vi "SCLN_TCPWritewithSize.vi"(8 "error in (no error)":errorcluster, 9 "timeout ms (600)":i32=25000, 10 "data in":string, 11 "connection ID":refnum<k5>) -> (0 "error out":errorcluster, 2 "bytes written":i32, 3 "connection ID out":refnum<k5>)   [LabVIEW 2015]
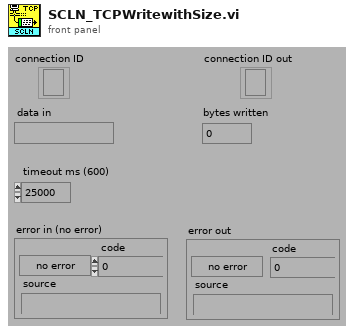
[diagram p1: front panel]
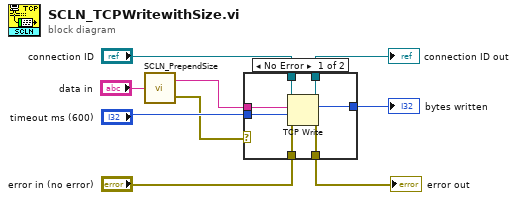
[diagram p0: block diagram]
diagram:
  n1 = call "SCLN_PrependSize.vi"("data"="data in") -> ("data with size"=w8:string, "error out"=w1:errorcluster)
  n2 = case shown="No Error" w1 {
    selector: w1 -> [_ w19]
    tunnel: w8 -> [w16 _]
    tunnel: "timeout ms (600)" -> [w15 w17]
    tunnel: "error in (no error)" -> [w14 _]
    tunnel: [w13 w19] -> w5
    tunnel: [w12 w17] -> w4
    tunnel: [w11 w18] -> w3
    tunnel: "connection ID" -> [w10 w18]
    frame No Error {
      n3 = TCP Write(connection ID=w10, data in=w16, error in (no error)=w14, 9:w15) -> (connection ID out=w11:refnum<k5>, bytes written=w12:i32, error out=w13:errorcluster)
    }
    frame Error {
    }
  }
  "bytes written" <- w4
  "connection ID out" <- w3
  "error out" <- w5
